vi "ResonanceAnalyzer.vi"() -> ()   [LabVIEW 2015]
uses:
  <vilib>/imath/engines/lvmath2/RunTimeEngine/Managers/WorkSpace/UID Generator.vi
  <vilib>/imath/engines/lvmath2/RunTimeEngine/ArithmeticOperatorToken/NIMS_ArithmeticOperator_power(S).vi
  <instcachedir>/0/NIMS_ArithmeticOperator_power(S)_DFB67823F1414E5097C86E39787D8CA8.lvgen/NIMS_ArithmeticOperator_power(S)_DFB67823F1414E5097C86E39787D8CA8_015.vi
  <vilib>/imath/engines/lvmath2/RunTimeEngine/RunTimeType/NIMS_RunTimeType_From StrictType (excl LVString).vi
  <instcachedir>/0/NIMS_RunTimeType_From StrictType (excl LVString)_EB1C38A9BC5048DA9ABDA8F781E54D21.lvgen/NIMS_RunTimeType_From StrictType (excl LVString)_EB1C38A9BC5048DA9ABDA8F781E54D21_000.vi
  <vilib>/imathl/engines/lvmath/Functions/Error Handling/Create Error.vi
  <vilib>/imath/engines/lvmath2/RunTimeEngine/LocalVariableDefStatement/MC_LocalVariableDefStatement_Display.vi
  <vilib>/imath/engines/lvmath2/RunTimeEngine/BuiltInFunctions/randnormal/NIMS_randnormal().vi
  <vilib>/imath/engines/lvmath2/RunTimeEngine/ErrorHandling/NIMS_Error From Error Code.vi
  <vilib>/imath/engines/lvmath2/RunTimeEngine/Managers/SymbolTable/Clear UID.vi
  <vilib>/imath/engines/lvmath2/RunTimeEngine/NodeEndStatement/NIMS_NodeEndStatement_Output.vi
  <instcachedir>/0/NIMS_NodeEndStatement_Output_53EC0D466D134D7ABD903AC30B43404B.lvgen/NIMS_NodeEndStatement_Output_53EC0D466D134D7ABD903AC30B43404B_009.vi
  <vilib>/imath/engines/lvmath2/RunTimeEngine/ErrorHandling/NIMS_Finalize Error.vi
  <vilib>/Utility/file.llb/Read Delimited Spreadsheet (DBL).vi
  <vilib>/gmath/NumericalOptimization/Nonlinear Curve Fit LM formula string.vi
  <vilib>/gmath/NI_Gmath.lvlib
  <vilib>/imath/engines/lvmath2/RunTimeEngine/Managers/SymbolTable/NIMS_WorkSpace.lvlib
panel:
  out "XY Graph":T1(graph)=[{"all rows"=[400.0, 405.0, 410.0, 415.0, 420.0, 425.0, 430.0, 435.0, 441.0, 446.0, 451.0, 456.0, 461.0, 466.0, 471.0, 476.0, 481.0, 486.0, 491.0, 496.0, 501.0, 506.0, 511.0, 516.0, 522.0, 527.0, 532.0, 537.0, 542.0, 547.0, 552.0, 557.0, 562.0, 567.0, 572.0, 577.0, 582.0, 587.0, 592.0, 597.0, 603.0, 608.0, 613.0, 618.0, 623.0, 628.0, 633.0, 638.0, 643.0, 648.0, 653.0, 658.0, 663.0, 668.0, 673.0, 678.0, 684.0, 689.0, 694.0, 699.0, 704.0, 709.0, 714.0, 719.0, 724.0, 729.0, 734.0, 739.0, 744.0, 749.0, 754.0, 759.0, 765.0, 770.0, 775.0, 780.0, 785.0, 790.0, 795.0, 800.0], "Best Gaussian Fit"=[0.10406402478738845, 0.11156709413884924, 0.11468131057567908, 0.13719099106598281, 0.13823902496857787, 0.13868209225119102, 0.12945473989176648, 0.13337825475540424, 0.1568251140579033, 0.16435425187572417, 0.16642620091243368, 0.1725196005592697, 0.1715272799569367, 0.19041480063378532, 0.18233689770570066, 0.20739499139216905, 0.21459347428327546, 0.22864559840659895, 0.24311532060683835, 0.24900583749740876, 0.27748804602627675, 0.2772526990268704, 0.31323225174550196, 0.3173600666612446, 0.34217692420981943, 0.3701755511370152, 0.3829401471632327, 0.40703914230712784, 0.45131583995927155, 0.474928909814884, 0.4955641984788935, 0.5442071687055933, 0.6086902002820426, 0.6685176890364458, 0.7270624496810163, 0.804071424186816, 0.8578716000146211, 0.9101439082698806, 0.9649796602172913, 0.9975810014795881, 0.986303120167285, 0.9668895090190252, 0.9163405311572789, 0.8531792635117502, 0.795822392742134, 0.7494239739727638, 0.6868352639845431, 0.6293041976054743, 0.5773230284373964, 0.5369359658540276, 0.5115083717997467, 0.4700733569200488, 0.46186649754245557, 0.4169267754147101, 0.3962613160263752, 0.3645498383063239, 0.35899213390006834, 0.3471067014107553, 0.3113290185761195, 0.3148268138291915, 0.3034243586199261, 0.27364050779934157, 0.26769276699277567, 0.2669269467115336, 0.28317252784167674, 0.24387248871508618, 0.22975421836547635, 0.2230052491981432, 0.2192161600646695, 0.20417523713610813, 0.19831796831407653, 0.20404258686496488, 0.187923108163129, 0.1995806852182272, 0.18015595656210498, 0.17845964692760527, 0.1901680673069202, 0.16882099660771824, 0.16359997658859893, 0.18707876363039813]}, {"all rows"=[400.0, 405.0, 410.0, 415.0, 420.0, 425.0, 430.0, 435.0, 441.0, 446.0, 451.0, 456.0, 461.0, 466.0, 471.0, 476.0, 481.0, 486.0, 491.0, 496.0, 501.0, 506.0, 511.0, 516.0, 522.0, 527.0, 532.0, 537.0, 542.0, 547.0, 552.0, 557.0, 562.0, 567.0, 572.0, 577.0, 582.0, 587.0, 592.0, 597.0, 603.0, 608.0, 613.0, 618.0, 623.0, 628.0, 633.0, 638.0, 643.0, 648.0, 653.0, 658.0, 663.0, 668.0, 673.0, 678.0, 684.0, 689.0, 694.0, 699.0, 704.0, 709.0, 714.0, 719.0, 724.0, 729.0, 734.0, 739.0, 744.0, 749.0, 754.0, 759.0, 765.0, 770.0, 775.0, 780.0, 785.0, 790.0, 795.0, 800.0], "Best Gaussian Fit"=[0.1187563159409578, 0.12265399115895585, 0.12674176192074357, 0.13103451535286287, 0.13554869328412866, 0.14030249749005597, 0.14531612764451116, 0.1506120580710166, 0.15737531691899248, 0.1633847812294103, 0.1697678811240875, 0.17656088724238794, 0.18380477045535878, 0.19154596353823924, 0.1998372693785834, 0.20873894764526862, 0.21832001925093839, 0.22865983695560674, 0.2398499812439429, 0.25199655313758934, 0.26522294941468094, 0.27967321941469664, 0.2955161129537899, 0.31294992893851203, 0.3363022797099644, 0.3581178629449344, 0.3824297435658715, 0.40963165252552003, 0.44018132689659983, 0.47460135005850684, 0.5134683471290101, 0.5573777835979186, 0.6068611814073064, 0.6622165290444273, 0.7231938611248109, 0.7884743211767369, 0.8549474855211208, 0.9170319299508402, 0.9667399911548693, 0.9954542264873535, 0.9945202572573685, 0.965201141813086, 0.9168582801764178, 0.8580286347640038, 0.7959790893260096, 0.7355182574928821, 0.6792189005796606, 0.6281195229995222, 0.5823698220621075, 0.5416721079143202, 0.505541585847466, 0.47344534912691744, 0.44486997895742936, 0.41935022675234623, 0.3964777206517084, 0.37590008873279823, 0.35381505406120184, 0.3372877342122649, 0.3222390880354791, 0.3084888589090492, 0.2958831086176947, 0.28428998872912253, 0.2735961932976033, 0.2637040035610606, 0.25452883383107133, 0.24599719542793566, 0.23804500637574733, 0.23061618580562804, 0.22366148236359526, 0.21713749492636725, 0.21100585152389037, 0.20523251865459521, 0.19873509228201933, 0.19364802638804934, 0.18883327669670644, 0.18426961239833392, 0.17993792533623387, 0.17582097511885778, 0.17190316951097273, 0.16817037463587825]}]
  out "Center Frequency":dbl=599.8514203984256
  out "Q":dbl=10.039683410144288
  in  "?":enum32{"Simulation", "Experiment"}(tab)=enum."Experiment"
  in  "End Frequency":dbl=800.0
  in  "Noise Level":dbl=0.01
  in  "df":dbl=5.0
  in  "Start Frequency":dbl=400.0
  in  "Center Frequency":dbl=600.0
  in  "Q":dbl=10.0
  in  "FIlename":path=path "C:/Users/mhsisk/week6/test.txt"
  in  "Best fit initial parameters":cluster{"Center Frequency":dbl, "Q":dbl}={"Center Frequency"=510.0, "Q"=10.0}
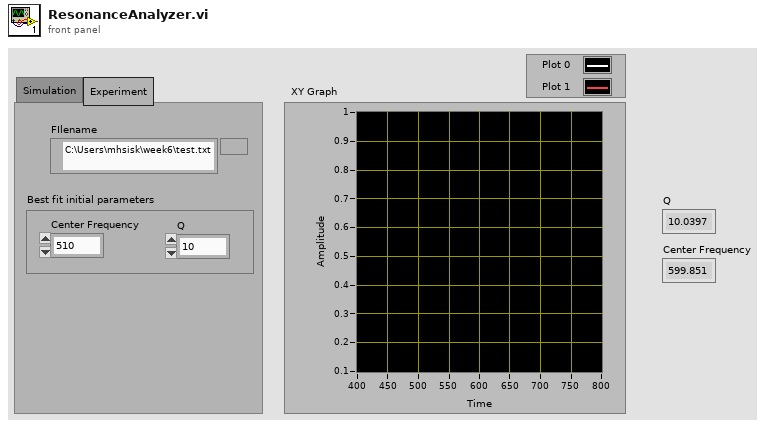
[diagram p1: front panel]
types:
  T1 = cluster{"all rows":dbl[], "Best Gaussian Fit":dbl[]}[]
  T2 = cluster{"model":string, "Parameters":string[], "x":string}
  T3 = cluster{"all rows":dbl[], "best nonlinear fit":dbl[]}
  T4 = cluster{"all rows":dbl[], "best nonlinear fit":cdb[]}[]
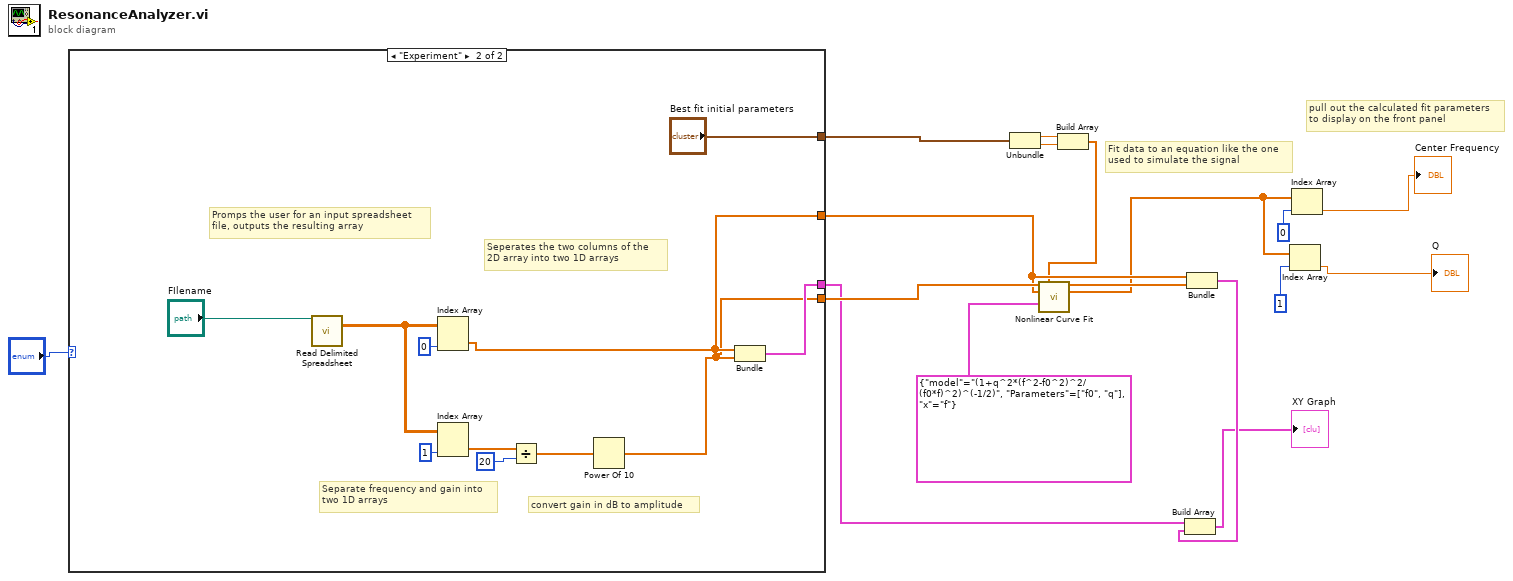
[diagram p0: block diagram]
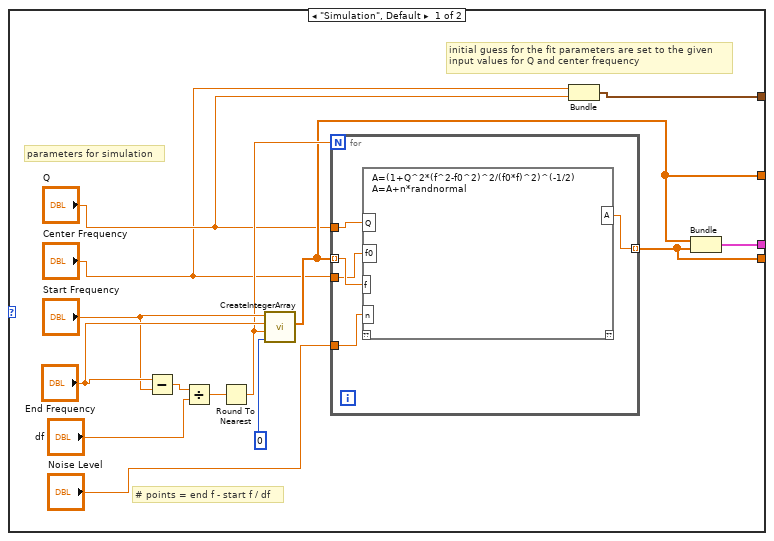
[diagram p2: hidden frame]
diagram:
  # "pull out the calculated fit parameters\nto display on the front panel"
  # "Fit data to an equation like the one\nused to simulate the signal"
  n1 = case shown="\"Experiment\"" "?" {
    tunnel: [w24 w138] -> w15
    tunnel: [w23 w139] -> w13
    tunnel: [w22 w140] -> w12
    tunnel: [w19 "Best fit initial parameters"] -> w1
    frame "Simulation", Default {
      # "initial guess for the fit parameters are set to the given \ninput values for Q and center frequency"
      # "parameters for simulation"
      # "# points = end f - start f / df"
      n2 = Subtract(x="End Frequency", y="Start Frequency") -> (x-y=w29:dbl)
      n3 = Divide(x=w29, y="df") -> (x/y=w26:dbl)
      n4 = Round To Nearest(number=w26) -> (nearest integer value=w25:dbl)
      n5 = call "CreateIntegerArray.vi"("Spacing"=0, "Number of Points"=w25, "Maximum"="End Frequency", "Minimum"="Start Frequency") -> ("Output Array"=w23:dbl[])  [unwired: 7 in]
      n6 = for {
        N: w25 -> [_]
        tunnel: "Center Frequency" -> [w34]
        tunnel: "Q" -> [w36]
        tunnel: w23 -> [w35] mode=indexing
        tunnel: [w33] -> w24 mode=indexing
        tunnel: "Noise Level" -> [w32]
        n7 = mathscript code="A=(1+Q^2*(f^2-f0^2)^2/(f0*f)^2)^(-1/2)\nA=A+n*randnormal"("Q"=w36, "f0"=w34, "f"=w35, "n"=w32) -> ("A"=w33:cdb)  [unwired: 1 in, 1 out]
      }
      n8 = Bundle("Center Frequency"="Center Frequency", "Q"="Q") -> (w19:cluster{"Center Frequency":dbl, "Q":dbl})  [unwired: 1 in]
      n9 = Bundle("Output Array"=w23, w24) -> (w22:cluster{"Output Array":dbl[], cdb[]})  [unwired: 1 in]
    }
    frame "Experiment" {
      # "convert gain in dB to amplitude"
      # "Separate frequency and gain into\ntwo 1D arrays"
      # "Seperates the two columns of the \n2D array into two 1D arrays"
      # "Promps the user for an input spreadsheet\nfile, outputs the resulting array"
      n10 = call-poly <vilib>:"Read Delimited Spreadsheet.vi"("file path (dialog if empty)"="FIlename") -> ("all rows"=w147:dbl[][])  [unwired: 9 in, 5 out]
      n11 = Index Array(array=w147, index (col)=0) -> (element=w139:dbl[])  [unwired: 1 in]
      n12 = Index Array(array=w147, index (col)=1) -> (element=w143:dbl[])  [unwired: 1 in]
      n13 = Divide(x=w143, y=20) -> (x/y=w141:dbl[])
      n14 = Power Of 10(x=w141) -> (10^x=w138:dbl[])
      n15 = Bundle("all rows"=w139, w138) -> (w140:cluster{"all rows":dbl[], dbl[]})  [unwired: 1 in]
    }
  }
  n16 = Unbundle(w1) -> ("Center Frequency"=w4:dbl, "Q"=w3:dbl)
  n17 = Build Array(w4, w3) -> (w2:dbl[])
  n18 = call-poly <vilib>:"Nonlinear Curve Fit.vi"("Y"=w15, "initial parameters"=w2, "X"=w13, "model description"=T2 {"model"="(1+q^2*(f^2-f0^2)^2/(f0*f)^2)^(-1/2)", "Parameters"=["f0", "q"], "x"="f"}) -> ("best nonlinear fit"=w14:dbl[], "best fit parameters"=w9:dbl[])  [unwired: 7 in, 3 out]
  n19 = Bundle("all rows"=w13, "best nonlinear fit"=w14) -> (w11:T3)  [unwired: 1 in]
  n20 = Build Array(w12, w11) -> (→"XY Graph":T4)
  n21 = Index Array(array=w9, index=1) -> (element=→"Q":dbl)
  n22 = Index Array(array=w9, index=0) -> (element=→"Center Frequency":dbl)
